vi "Terminate.vi"(8 "error in (no error)":errorcluster, 10 "Message in":refnum<class "TerminateMessage.lvclass">, 11 "ExampleClassC in":refnum<class "ExampleClassC.lvclass">) -> (0 "error out":errorcluster, 3 "ExampleClassC out":refnum<class "ExampleClassC.lvclass">)   [LabVIEW 2012, in "ExampleClassC.lvclass"]
doc: "This member function is called when the statemachine in the run.vi receives an 'terminate' command. It closes the RabbitMQ connection. \n\nOverride this member function in your derived class to release all previously acquired resources (but don't forget to call the parent method). If your component has subcomponents, they count as resources, and you have to release them by calling their own terminate functions."
uses:
  ExampleClassC.lvclass
  <vilib>/Distrio/Murmex/TerminateMessage/TerminateMessage.lvclass
  <vilib>/Distrio/Murmex/Murmex/Murmex.lvclass
panel:
  # "This method is called when the TERMINATE\ntrigger is sent. \n\nOverride this method when your component needs to\nrespond to this trigger. \n\nCall parent for proper implementation"
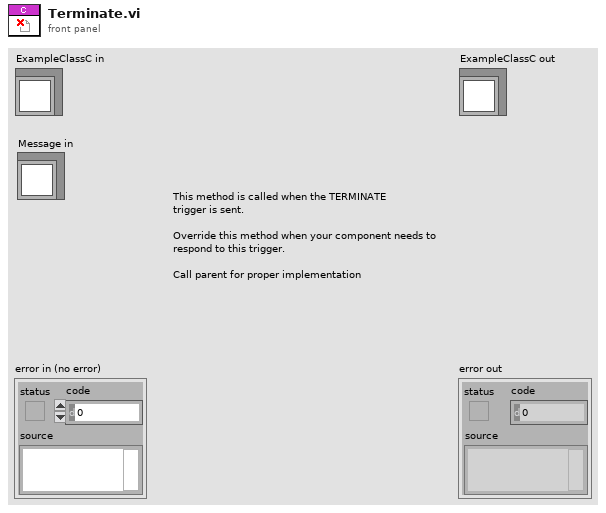
[diagram p1: front panel]
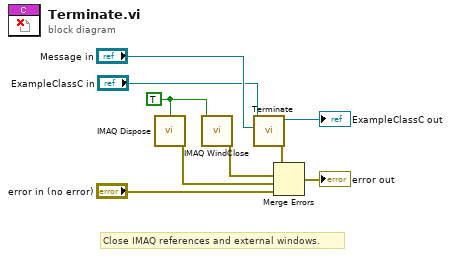
[diagram p0: block diagram]
diagram:
  w8 = TRUE ("All Images? (No)")
  # "Close IMAQ references and external windows."
  n1 = call "IMAQ Dispose"("All Images? (No)"=w8) -> ("error out"=w1:errorcluster)  [unwired: 5 in]
  n2 = call "IMAQ WindClose"("Close All Windows (False)"=w8) -> ("error out"=w2:errorcluster)  [unwired: 5 in]
  n3 = call-parent "Terminate.vi"("Message in"="Message in", "Murmex in"="ExampleClassC in") -> ("error out"=w5:errorcluster, "Murmex out"=→"ExampleClassC out":refnum<class "ExampleClassC.lvclass">)  [unwired: 8 in]
  n4 = Merge Errors(w5, w2, w1, "error in (no error)") -> (→"error out":errorcluster)
